vi "Put msg in mailbox.vi"(8 "error in (no error)":errorcluster, 10 "Message":T1 {"Time Stamp" format="%<%H:%M:%S\n%Y/%m/%d>T"}, 11 "Mailbox ref in":T2) -> (0 "error out":errorcluster, 2 "timed out?":bool, 3 "mailbox ref out":T2)   [LabVIEW 2021, in "Queued messenger.lvlib"]
doc: "Puts any message to mailbox. The message will be converted to variant. (Recomended to use general message.)"
uses:
  <userlib>/MatS libs/MatS Messenger/Queued messenger.lvlib
  <userlib>/MatS libs/MatS Messenger/TypeDefs/Mailbox ref.ctl
  <userlib>/MatS libs/MatS Messenger/TypeDefs/General message.ctl
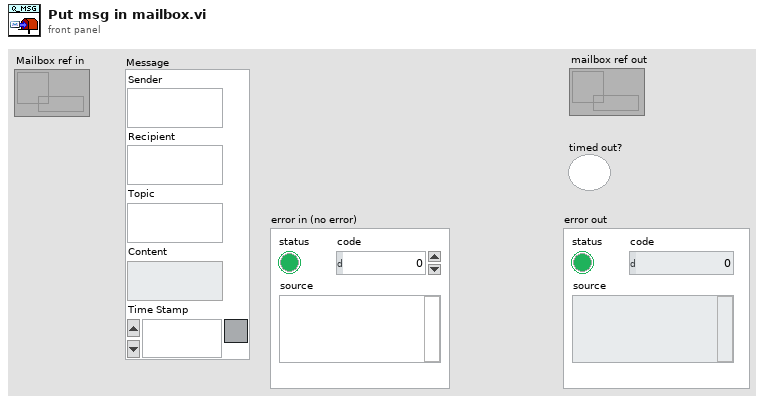
[diagram p1: front panel]
types:
  T1 = typedef "Queued messenger.lvlib/General message.ctl" = cluster{"Sender":string, "Recipient":string, "Topic":string, "Content":variant, "Time Stamp":timestamp}
  T2 = typedef "Queued messenger.lvlib/Mailbox ref.ctl" = refnum<queue>
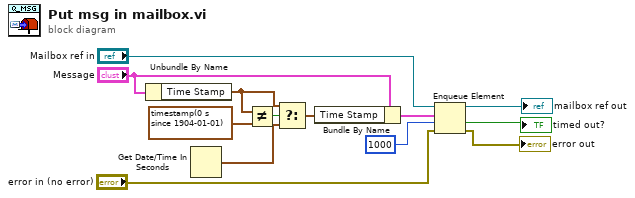
[diagram p0: block diagram]
diagram:
  n1 = Unbundle By Name("Message") -> ("Time Stamp"=w4:timestamp)
  n2 = Get Date/Time In Seconds() -> (seconds since 1Jan1904=w3:timestamp)
  n3 = Not Equal?(x=w4, y=timestamp(0 s since 1904-01-01) ("Time Stamp")) -> (x != y?=w5:bool)
  n4 = Select(t=w4, s=w5, f=w3) -> (s? t:f=w1:timestamp)
  n5 = Bundle By Name(cluster="Message", "Time Stamp"=w1) -> (w2:T1)
  n6 = Enqueue Element(queue="Mailbox ref in", element=w2, timeout in ms (-1)=1000, error in (no error)="error in (no error)") -> (queue out=→"mailbox ref out":T2, timed out?=→"timed out?":bool, error out=→"error out":errorcluster)
